vi "_36_Sample_qsns_9[12].vi"() -> ()   [LabVIEW 2020]
panel:
  out "offset past match":i32
  out "after substring":string
  out "match substring":string
  out "before substring":string
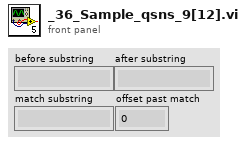
[diagram p1: front panel]
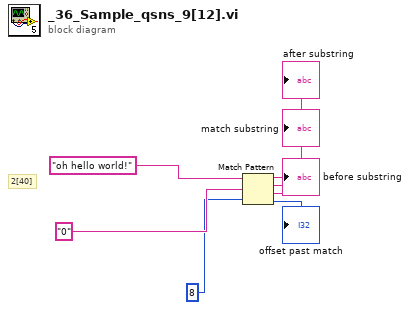
[diagram p0: block diagram]
diagram:
  # "2[40]"
  n1 = Match Pattern(string="oh hello world!", regular expression="0", offset (0)=8) -> (before substring=→"before substring":string, match substring=→"match substring":string, after substring=→"after substring":string, offset past match=→"offset past match":i32)
